vi "Wait.vi"(8 "error in (no error)":errorcluster, 10 "Params":variant, 11 "NI SMU in":refnum<class "NI SMU.lvclass">) -> (0 "error out":errorcluster, 3 "NI SMU out":refnum<class "NI SMU.lvclass">)   [LabVIEW 2020, in "NI SMU.lvlib" / "NI SMU.lvclass"]
uses:
  NI SMU.lvclass
  NI SMU.lvclass/NI SMU.ctl
  <instrlib>/niDCPower/nidcpower.llb/niDCPower Wait For Event - Event.ctl
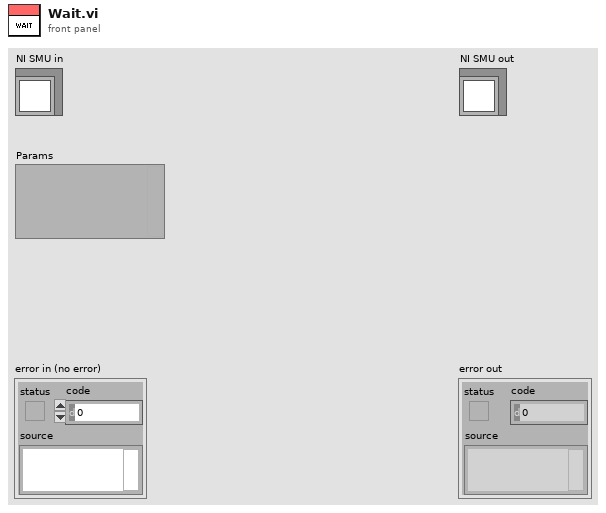
[diagram p1: front panel]
types:
  T1 = typedef "niDCPower Wait For Event - Event.ctl" = i32
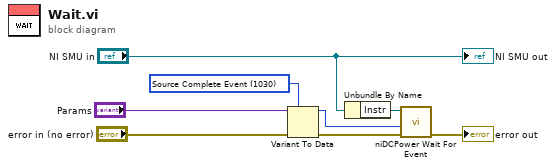
[diagram p0: block diagram]
diagram:
  w6 = T1 1030 items=["Source Complete Event"=1030, "Measure Complete Event"=1031, "Sequence Iteration Complete Event"=1032, "Sequence Engine Done Event"=1033, "Pulse Complete Event"=1051, "Ready For Pulse Trigger Event"=1052] ("event")
  n1 = Variant To Data(error in="error in (no error)", type=w6, Variant="Params") -> (data=w5:T1, error out=w7:errorcluster)
  n2 = Unbundle By Name("NI SMU in") -> ("Instr"=w8:refnum<k15>)
  n3 = call <instrlib>:"niDCPower Wait For Event.vi"("error in (no error)"=w7, "event"=w5, "instrument handle"=w8) -> ("error out"=→"error out":errorcluster)  [unwired: 7 in, 1 out]
  "NI SMU out" <- "NI SMU in"
